vi "Set All Minimum Log Level.vi"(8 "error in":errorcluster, 11 "log level (Info)":T1=enum."Info") -> (0 "error out":errorcluster)   [LabVIEW 2018, in "GLog.lvlib"]
doc: "Set the minimum log level of all actively registered loggers in the Registry."
uses:
  GLog.lvlib
  logger_class/Log Levels.ctl
  registry/Registry.lvlib
  logger_class/Logger.lvclass
panel:
  # "Connector Pane"
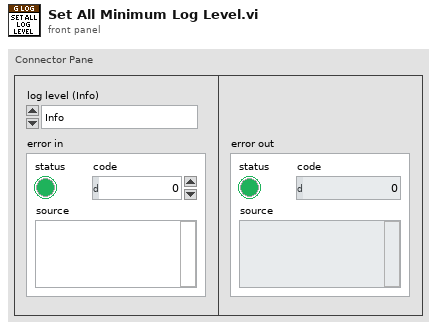
[diagram p1: front panel]
types:
  T1 = typedef "GLog.lvlib/Logger.lvclass/Log Levels.ctl" = enum16{"Trace", "Debug", "Info", "Warning", "Error", "Critical"}
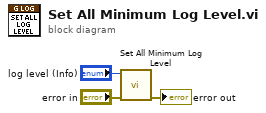
[diagram p0: block diagram]
diagram:
  n1 = call "Set All Minimum Log Level.vi"("error in"="error in", "log level"="log level (Info)") -> ("error out"=→"error out":errorcluster)  [unwired: 9 in]
